vi "String.vi"() -> ()   [LabVIEW 2018]
panel:
  out "결과 문자열":string
  in  "초기 문자열":string
  out "부분 문자열":string
  out "문자열 3":string
  in  "문자열 2":string
  in  "문자열":string
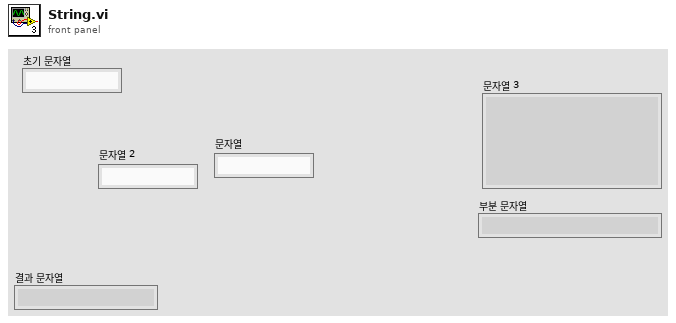
[diagram p1: front panel]
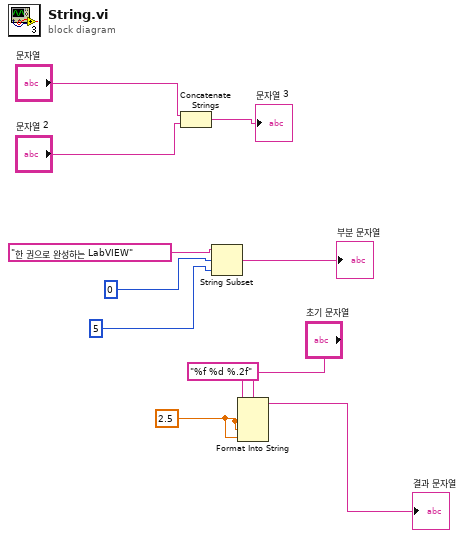
[diagram p0: block diagram]
diagram:
  w3 = 2.5
  n1 = Concatenate Strings("문자열", "문자열 2") -> (→"문자열 3":string)
  n2 = String Subset(string="한 권으로 완성하는 LabVIEW", offset (0)=0, length (rest)=5) -> (substring=→"부분 문자열":string)
  n3 = Format Into String(format string="%f %d %.2f" ("포맷 문자열"), initial string="초기 문자열", w3, w3, w3) -> (resulting string=→"결과 문자열":string)  [unwired: 1 in, 1 out]
